vi "TreeNode Get Segment.vi"(8 "error in (no error)":errorcluster, 10 "Segment index":i32, 11 "TreeNode DVR in":refnum<data-value>) -> (0 "error out":errorcluster, 2 "Data out":refnum<data-value>, 3 "TreeNode DVR out":refnum<data-value>)   [LabVIEW 2012, in "MDSplus.lvlib"]
doc: "Get data form the selected segment."
uses:
  <vilib>/MDSplus/Library/MDSplus.lvlib
  <vilib>/MDSplus/Classes/Data_Class/TreeNode_Class/TreeNode.lvclass
  <vilib>/MDSplus/Classes/Data_Class/Array_Class/Array.lvclass
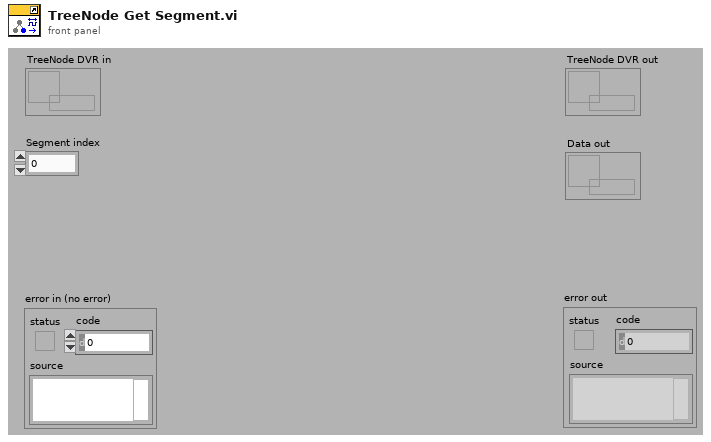
[diagram p1: front panel]
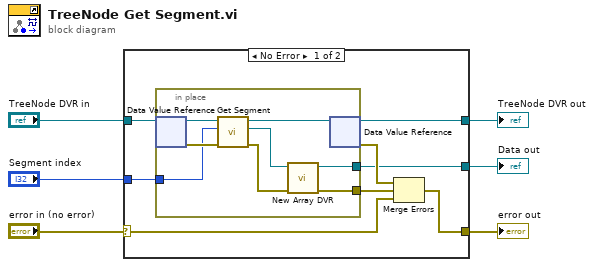
[diagram p0: block diagram]
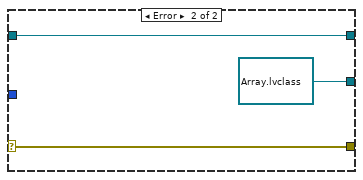
[diagram p2: hidden frame]
diagram:
  n1 = case shown="No Error" "error in (no error)" {
    selector: "error in (no error)" -> [w13 w25]
    tunnel: "TreeNode DVR in" -> [w14 w24]
    tunnel: [w10 w25] -> w6
    tunnel: [w11 w24] -> w3
    tunnel: [w8 refnum<data-value> refnum ("Data DVR")] -> w2
    tunnel: "Segment index" -> [w7 _]
    frame No Error {
      n2 = in-place {
        in-place-border: [w18] -> w8
        in-place-border: [w17] -> w9
        in-place-border: w7 -> [w15]
        n3 = in-place-dvr #1(w14) -> (w22:refnum<class "TreeNode.lvclass">, w21:errorcluster)
        n4 = call-dynamic "Get Segment.vi"("error in (no error)"=w21, "Segment index"=w15, "TreeNode in"=w22) -> ("error out"=w16:errorcluster, "Data out"=w19:refnum<class "Array.lvclass">, "TreeNode out"=w20:refnum<class "TreeNode.lvclass">)  [unwired: 6 in]
        n5 = call <vilib>:"New Array DVR.vi"("error in (no error)"=w16, "Array in"=w19) -> ("error out"=w17:errorcluster, "Array DVR out"=w18:refnum<data-value>)  [unwired: 8 in]
        n6 = in-place-dvr #1(w20) -> (w11:refnum<data-value>, w12:errorcluster)
      }
      n7 = Merge Errors(w12, w9, w13) -> (w10:errorcluster)
    }
    frame Error {
    }
  }
  "error out" <- w6
  "TreeNode DVR out" <- w3
  "Data out" <- w2
